vi "main.vi"() -> ()   [LabVIEW 2019]
uses:
  <vilib>/express/express analysis/Spectral/Block/exnSpectralBlock spectral measurements peak poly.vi
  <vilib>/express/express analysis/Spectral/Block/exnSpectralBlock spectral measurements peak DDT.vi
  <vilib>/express/express analysis/Spectral/XNode/ExpressSpectralMeasurementsBlockNode.xnode
panel:
  in  "Knob":dbl(knob) scale=0.1..10.0
  out "Thermometer":dbl(slide) scale=0.0..10.0
  out "Peak to Peak":dbl
  in  "nr har 2":dbl
  in  "f":dbl(knob) min=0.0 max=100.0 scale=0.0..50.0
  in  "amp2":dbl(knob) scale=0.0..10.0
  in  "amp1":dbl(knob) scale=0.0..10.0
  in  "Tab Control":enum32{"Page 1", "Page 2", "Page 3", "Page 4"}(tab)
  out "Waveform Graph":dynamicdata(graph)
  out "Waveform Chart":dynamicdata(graph)
  out "Waveform Graph 2":dynamicdata(graph)
  out "Waveform Graph 3":dynamicdata(graph)
  out "x+1":i32
  in  "stop":bool
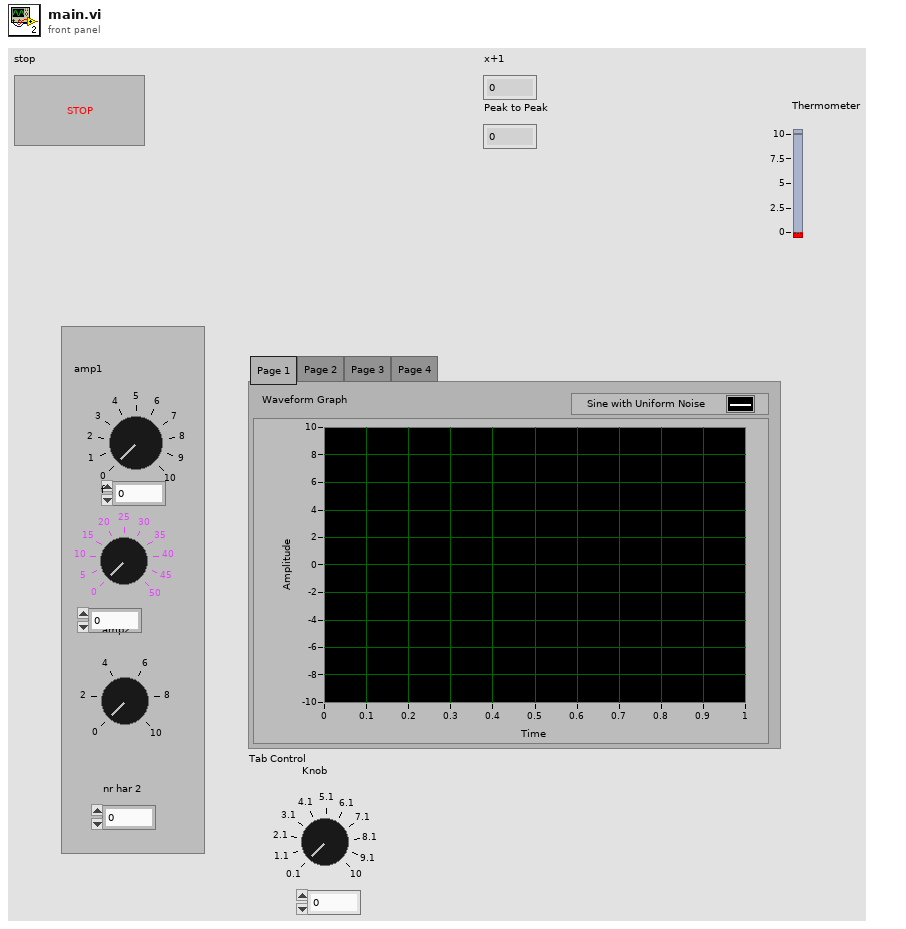
[diagram p1: front panel]
types:
  T1 = cluster{"averaging mode":u16, "weighting mode":u16, "number of averages":u32}
  T2 = cluster{"dB On (F)":bool, "unwrap phase (F)":bool, "convert to degree (F)":bool}
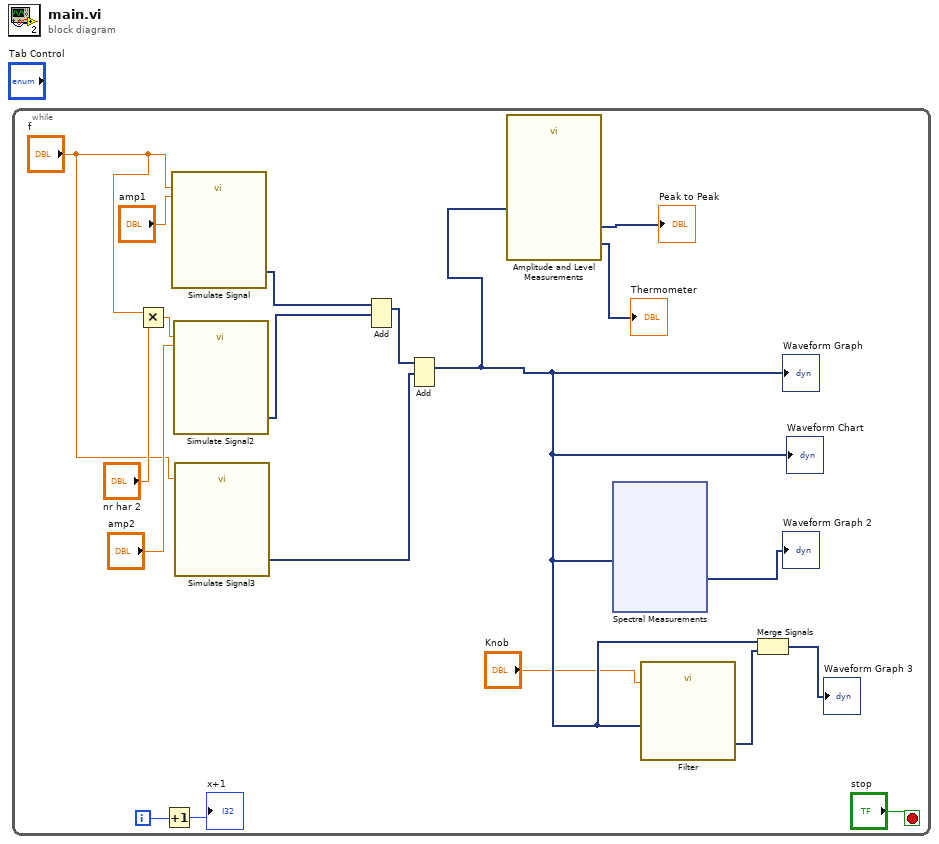
[diagram p0: block diagram]
diagram:
  n1 = while {
    i -> [w18]
    stop <- "stop" stop-if-true
    n2 = Multiply(x="f", y="nr har 2") -> (x*y=w9:dbl)
    n3 = Increment(x=w18) -> (x+1=→"x+1":i32)
    n4 = call "Simulate Signal"("Frequency"="f", "Amplitude"="amp1") -> ("Sine with Uniform Noise"=w16:dynamicdata)  [unwired: 12 in, 1 out]
    n5 = call "Simulate Signal2"("Frequency"=w9, "Amplitude"="amp2") -> ("Sine"=w15:dynamicdata)  [unwired: 12 in, 1 out]
    n6 = call "Simulate Signal3"("Frequency"="f") -> ("Sine"=w13:dynamicdata)  [unwired: 13 in, 1 out]
    n7 = Add(1:w15, 2:w16) -> (0:w14:dynamicdata)  [unwired: 1 in, 1 out]
    n8 = Add(1:w13, 2:w14) -> (0:w4:dynamicdata)  [unwired: 1 in, 1 out]
    "Waveform Graph" <- w4
    "Waveform Chart" <- w4
    n9 = call "Amplitude and Level Measurements"("Signals"=w4) -> ("RMS"=→"Thermometer":dynamicdata, "Peak to Peak"=→"Peak to Peak":dynamicdata)  [unwired: 12 in, 1 out]
    n10 = xnode "Spectral Measurements"("Signals"=w4) -> ("FFT - (Peak)"=→"Waveform Graph 2":dynamicdata)  [unwired: 1 in, 2 out]
    n11 = call "Filter"("Lower Cut-Off"="Knob", "Signal"=w4) -> ("Filtered Signal"=w3:dynamicdata)  [unwired: 8 in, 1 out]
    n12 = Merge Signals(w4, w3) -> (→"Waveform Graph 3":dynamicdata)
  }
